vi "Agilent_value_set.vi"(1 "Current (A)":dbl) -> ()   [LabVIEW 2017]
panel:
  out "VISA resource name out":refnum<visa-resource-name>
  in  "VISA resource name":refnum<visa-resource-name>
  out "error out":errorcluster
  in  "error in (no error)":errorcluster
  in  "cycle_count":i32
  in  "delay":i32
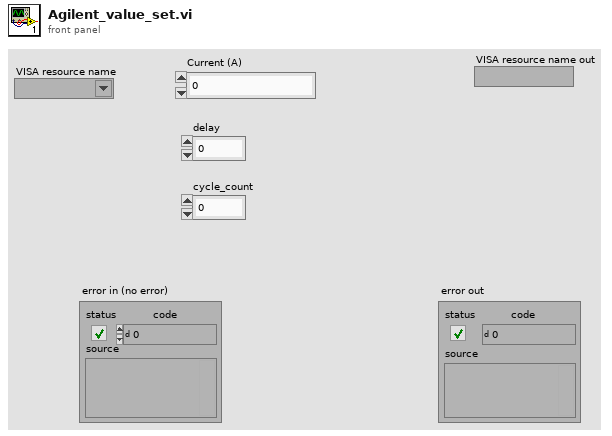
[diagram p1: front panel]
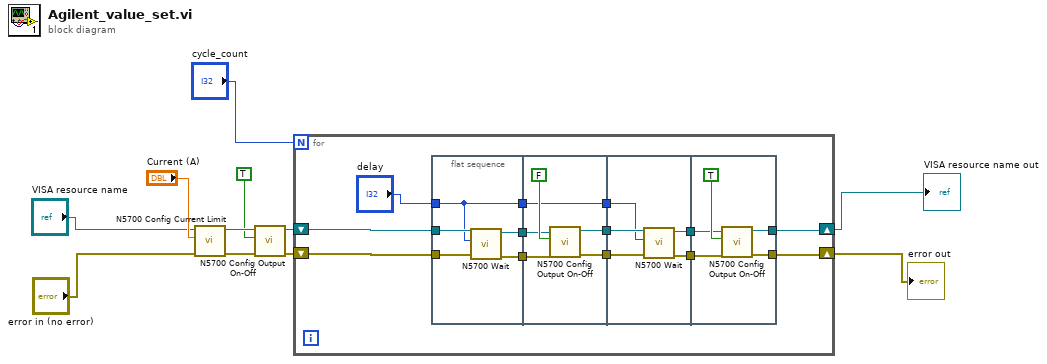
[diagram p0: block diagram]
diagram:
  n1 = call <instrlib>:"N5700 Config Current Limit.vi"("error"="error in (no error)", "Current Limit"="Current (A)", "VISA"="VISA resource name") -> ("error out"=w9:errorcluster, "VISA out"=w7:refnum<visa-resource-name>)  [unwired: 4 in]
  n2 = call <instrlib>:"N5700 Config Output On-Off.vi"("error"=w9, "Output ON"=TRUE, "VISA"=w7) -> ("error out"=w10:errorcluster, "VISA out"=w8:refnum<visa-resource-name>)  [unwired: 4 in]
  n3 = for {
    N: "cycle_count" -> [_]
    shift-right: [w16] -> w4
    shift-left: w8 -> [w18]
    shift-right: [w15] -> w3
    shift-left: w10 -> [w17]
    n4 = flat-sequence {
      tunnel: [w29] -> w24
      tunnel: [w28] -> w23
      tunnel: w18 -> [w27]
      tunnel: w17 -> [w26]
      tunnel: "delay" -> [w25]
      tunnel: [w25] -> w13
      tunnel: w24 -> [w34]
      tunnel: w23 -> [w33]
      tunnel: [w32] -> w22
      tunnel: [w31] -> w21
      tunnel: [w30] -> w14
      tunnel: w13 -> [w30]
      tunnel: w22 -> [w40]
      tunnel: w21 -> [w39]
      tunnel: [w38] -> w20
      tunnel: [w37] -> w19
      tunnel: w14 -> [w36]
      tunnel: w20 -> [w43]
      tunnel: w19 -> [w44]
      tunnel: [w42] -> w16
      tunnel: [w41] -> w15
      frame #0 {
        n5 = call <instrlib>:"N5700 Wait.vi"("error"=w26, "Delay (20 mS)"=w25, "VISA"=w27) -> ("error out"=w28:errorcluster, "VISA out"=w29:refnum<visa-resource-name>)  [unwired: 4 in]
      }
      frame #1 {
        n6 = call <instrlib>:"N5700 Config Output On-Off.vi"("error"=w33, "Output ON"=FALSE, "VISA"=w34) -> ("error out"=w31:errorcluster, "VISA out"=w32:refnum<visa-resource-name>)  [unwired: 4 in]
      }
      frame #2 {
        n7 = call <instrlib>:"N5700 Wait.vi"("error"=w39, "Delay (20 mS)"=w36, "VISA"=w40) -> ("error out"=w38:errorcluster, "VISA out"=w37:refnum<visa-resource-name>)  [unwired: 4 in]
      }
      frame #3 {
        n8 = call <instrlib>:"N5700 Config Output On-Off.vi"("error"=w43, "Output ON"=TRUE, "VISA"=w44) -> ("error out"=w41:errorcluster, "VISA out"=w42:refnum<visa-resource-name>)  [unwired: 4 in]
      }
    }
  }
  "error out" <- w3
  "VISA resource name out" <- w4
